vi "Factorial of a give number using for loop.vi"() -> ()   [LabVIEW 2024]
panel:
  out "Output":dbl
  in  "Constant":dbl
  in  "Count":dbl
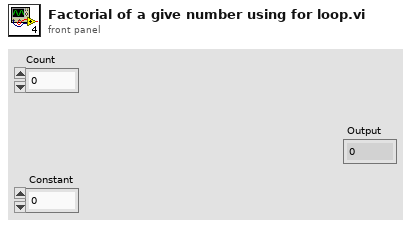
[diagram p1: front panel]
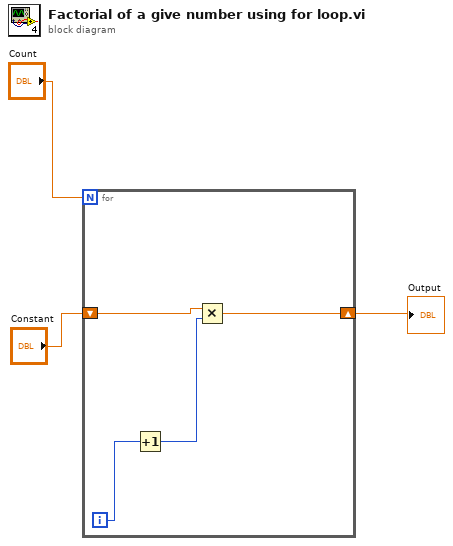
[diagram p0: block diagram]
diagram:
  n1 = for {
    N: "Count" -> [_]
    shift-right: [w7] -> w3
    shift-left: "Constant" -> [w6]
    i -> [w4]
    n2 = Increment(x=w4) -> (x+1=w5:i32)
    n3 = Multiply(x=w6, y=w5) -> (x*y=w7:dbl)
  }
  "Output" <- w3
